vi "New Style Object.vi"(8 "error in (no error)":errorcluster, 10 "Font":T1={"Name"="Calibri", "Size"=12, "Bold"=FALSE, "Italic"=FALSE, "Underline"=18, "Strike"=FALSE, "Color"=0, "Alignment"=1} {"Alignment" items=["LEFT"=1, "CENTER"=2, "RIGHT"=3, "BOTH"=4, "MEDIUM_KASHIDA"=5, "DISTRIBUTE"=6, "NUM_TAB"=7, "HIGH_KASHIDA"=8, "LOW_KASHIDA"=9, "THAI_DISTRIBUTE"=10]; "Underline" items=["Single"=1, "Words"=2, "Double"=3, "Thick"=4, "Dotted"=5, "DottedHeavy"=6, "Dash"=7, "DashedHeavy"=8, "DashLong"=9, "DashLongHeavy"=10, "DotDash"=11, "DashDotHeavy"=12, "DotDotDash"=13, "DashDotDotHeavy"=14, "Wave"=15, "WavyHeavy"=16, "WavyDouble"=17, "None"=18]}, 11 "Style Name":string="Default") -> (0 "error out":errorcluster, 3 "Style out":refnum<class "Style.lvclass">)   [LabVIEW 2020, in "Styles.lvlib" / "Style.lvclass"]
uses:
  Style.lvclass
  Font--cluster.ctl
  Underline--ring.ctl
  Alignment--ring.ctl
  Style.lvclass/Style.ctl
  Set Style Name.vi
  Styles.lvlib
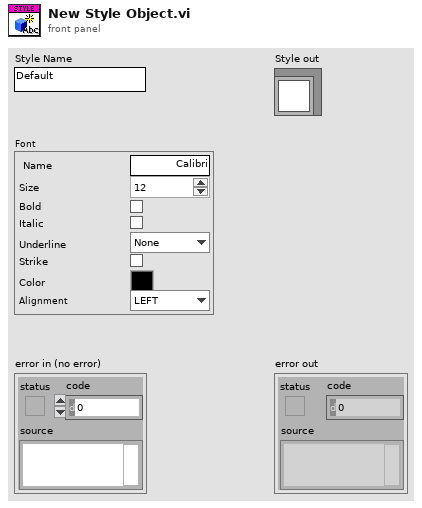
[diagram p1: front panel]
types:
  T1 = typedef "Styles.lvlib/Font--cluster.ctl" = cluster{"Name":string, "Size":i32, "Bold":bool, "Italic":bool, "Underline":T2, "Strike":bool, "Color":u32, "Alignment":T3}
  T2 = typedef "Styles.lvlib/Underline--ring.ctl" = i32
  T3 = typedef "Styles.lvlib/Alignment--ring.ctl" = i32
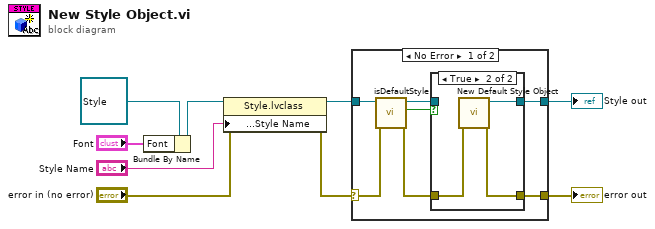
[diagram p0: block diagram]
diagram:
  n1 = Bundle By Name(cluster=refnum<class "Style.lvclass"> refnum ("Font in"), "Font"="Font") -> (w2:refnum<class "Style.lvclass">)
  n2 = property class="Style.lvclass"(reference=w2, error in="error in (no error)", "Public VIs:Properties:Style Name"="Style Name") -> (reference out=w6:refnum<class "Style.lvclass">, error out=w3:errorcluster)
  n3 = case shown="No Error" w3 {
    selector: w3 -> [w15 w23]
    tunnel: w6 -> [w16 w22]
    tunnel: [w12 w22] -> w8
    tunnel: [w10 w23] -> w7
    frame No Error {
      n4 = call-dynamic "isDefaultStyle.vi"("error in (no error)"=w15, "Style in"=w16) -> ("error out"=w11:errorcluster, "isDefault"=w13:bool, "Style out"=w14:refnum<class "Style.lvclass">)  [unwired: 7 in]
      n5 = case shown="True" w13 {
        tunnel: w14 -> [w18 _]
        tunnel: [w18 w21] -> w12
        tunnel: w11 -> [w17 w20]
        tunnel: [w17 w19] -> w10
        frame False {
        }
        frame True {
          n6 = call "New Default Style Object.vi"("error in (no error)"=w20) -> ("error out"=w19:errorcluster, "Style out"=w21:refnum<class "Style.lvclass">)  [unwired: 9 in]
        }
      }
    }
    frame Error {
    }
  }
  "error out" <- w7
  "Style out" <- w8
